vi "Main UI.vi"() -> ()   [LabVIEW 2017, in "Example UI.lvlib"]
uses:
  Example UI.lvlib
  CBTF Modules/Classes/Application/Class/typedefs/Test Info -- Cluster.ctl
  <vilib>/TSS/ACRObat Test Framework/Core Launcher/Core Manager Methods -- Enum.ctl
  <vilib>/TSS/ACRObat Test Framework/Utilities/User Manager/User Manager.Base/typedefs/User Groups -- Enum.ctl
  <vilib>/TSS/ACRObat Test Framework/Classes/Data/Data Viewer/Class/Data Viewer.lvclass
  C:/Program Files (x86)/National Instruments/LabVIEW 2017/vi.lib/TSS/ACRObat Test Framework/Classes/Base Objects/Base Class/Base Class/Base Class.lvclass
  CBTF Modules/Classes/Application/Class/typedefs/Op Mode -- Enum.ctl
  Application/Class/Example Application.lvclass
  C:/Test System Services/Acrobat Framework/CBTF Modules/Classes/Application/Class/Application.lvclass
  <vilib>/Utility/miscctls.llb/LVRowAndColumnTypeDef.ctl
  Application/Properties/DUT State -- Enum.ctl
  CBTF Modules/Classes/Test Recipe/Class/Test Recipe.lvclass
  CBTF Modules/Classes/Application/Class/Public API/Settings/Adjust Application Settings.vi
  <vilib>/TSS/ACRObat Test Framework/Utilities/User Manager/User Manager.FileDB/User Library.FileDB.lvclass
  <vilib>/TSS/ACRObat Test Framework/Classes/Data/Data Logger/Class/Data Logger.lvclass
  <vilib>/TSS/ACRObat Test Framework/Core Launcher/Core Launcher.lvlib
  <vilib>/TSS/ACRObat Test Framework/Classes/Base Objects/Base Class/Base Class/Base Class.lvclass
  CBTF Modules/Classes/Application/Class/Application.lvclass
  <vilib>/TSS/ACRObat Test Framework/Utilities/User Manager/User Manager.Base/User Library.Base.lvclass
  Application/Properties/Example App Properties.lvclass
  <vilib>/TSS/ACRObat Test Framework/Classes/Data/Data Repo/Class/Data Repo.lvclass
panel:
  out "Gold Board":bool
  in  "Iterations":u32=1
  in  "Serial 6":string caption="Serial ID 6"
  in  "Status 6":string
  in  "Serial 5":string caption="Serial ID 5"
  in  "Status 5":string
  in  "Serial 4":string caption="Serial ID 4"
  in  "Status 4":string
  in  "Settings":bool
  out "VER":bool
  out "ENG":bool
  in  "Serial 3":string caption="Serial ID 3"
  in  "Status 3":string
  in  "Serial 2":string caption="Serial ID 2"
  in  "Status 2":string
  in  "Serial 1":string caption="Serial ID 1"
  in  "Status 1":string
  in  "User Login":bool
  out "Results":i32(listbox)=-1
  in  "Test Information":T1
  in  "Run":bool
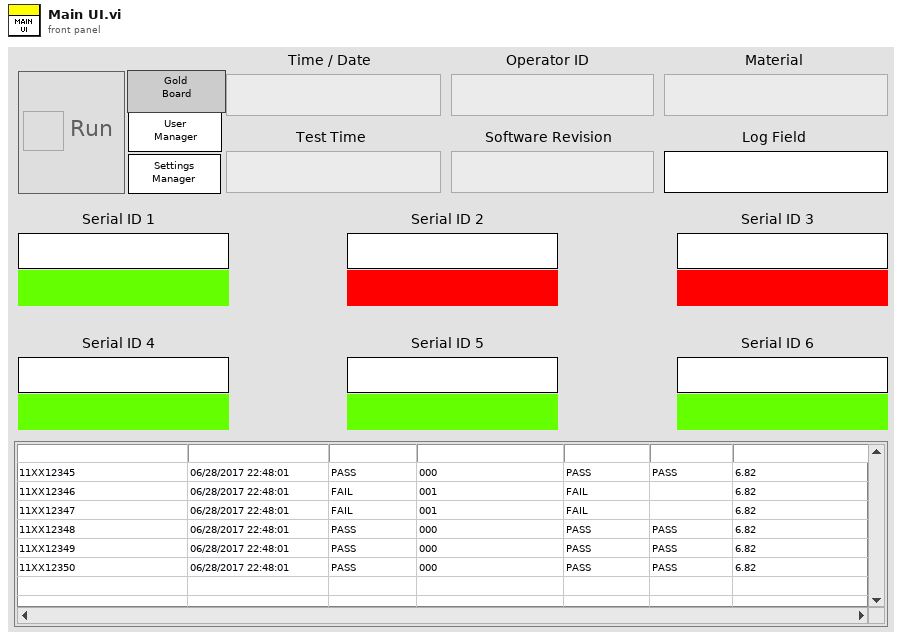
[diagram p1: front panel]
types:
  T1 = typedef "Application.lvlib/Application.lvclass/Test Info -- Cluster.ctl" = cluster{"Time / Date":string, "Operator ID":string, "Material":string, "Log Field":string, "Test Time":string, "Software Revision":string}
  T2 = typedef "Core Launcher.lvlib/Core Manager Methods -- Enum.ctl" = enum16{"Spawn Objects", "Get Objects", "Destroy Objects"}
  T3 = typedef "Utilities.lvlib/User Library.Base.lvclass/User Groups -- Enum.ctl" = enum16{"unknown", "Standard", "Engineering", "Super"}
  T4 = enum32{"invalid app kind", "Development System", "Run Time System", "Student Edition", "Embedded LabVIEW", "Evaluation", "Custom"}
  T5 = typedef "LVRowAndColumnTypeDef.ctl" = cluster{"Row":i32, "Column":i32}
  T6 = enum8{"Enabled", "Disabled", "Disabled and Grayed Out"}
  T7 = enum32{"Invalid", "Standard", "Closed", "Hidden", "Minimized", "Maximized"}
  T8 = enum16{"Idle", "Ready", "Running Test", "Paused"}
  T9 = typedef "Example Application.lvlib/Example App Properties.lvclass/DUT State -- Enum.ctl" = enum16{"Idle", "Ready", "Testing", "Passed", "Failed"}
  T10 = typedef "eventvkey.ctl" = enum16{"ASCII", "Enter", "Return", "Shift", "Ctrl", "Alt", "Cmd", "Opt", "Caps", "NumLock", "Clear", "Break", "Up", "Down", "Left", "Right", "Insert", "Delete", "Home", "End", "PageUp", "PageDown", "Escape", "Help", "Pause", "ScrollLock", "F1", "F2", "F3", "F4", "F5", "F6", "F7", "F8", "F9", "F10", "F11", "F12", "F13", "F14", "F15", "F16", "F17", "F18", "F19", "F20", "F21", "F22", "F23", "F24", "Play", "VolumeUp", "VolumeDown", "Mute", "Two Byte Char"}
  T11 = typedef "Application.lvlib/Application.lvclass/Op Mode -- Enum.ctl" = u16
  T12 = cluster{"Core":cluster{"Current VI Reference":refnum<vi>, "Close Panel on Exit?":bool}, "Application":refnum<class "Example Application.lvclass">, "Data Viewer":refnum<class "Data Viewer.lvclass">, "Op Mode":T11, "Current UUT":i16, "UI State":enum16{"Idle", "Ready", "Running Test", "Paused"}, "Tick Count":u64}
  T13 = cluster{"Current VI Reference":refnum<vi>, "Close Panel on Exit?":bool}
  T14 = typedef "Application.lvlib/App Properties.lvclass/Class Properties -- Cluster.ctl" = cluster{"UUT Info":T15[], "Test Information":refnum<vi>, "Gold Board":refnum<class "Golden Board.lvclass">, "Test Recipe":refnum<class "Test Recipe.lvclass">, "Instruments":refnum<class "Instrument.lvclass">[], "Mode":T11, "Test Results":T16[], "Station Config":refnum<class "Station Config.lvclass">, "Variable Engine":refnum<class "Variable Engine.lvclass">}
  T15 = typedef "Application.lvlib/App Properties.lvclass/UUT Reference -- Cluster.ctl" = cluster{"Serial Number Reference":refnum<vi>, "Status Message Reference":refnum<vi>}
  T16 = typedef "Application.lvlib/App Properties.lvclass/Test Result -- Cluster.ctl" = cluster{"Position":i32, "Pass":bool, "Fail Codes":string}
  T17 = typedef "Data Logger.lvlib/Data Logger Settings.lvclass/Class Settings -- Cluster.ctl" = cluster{"Mode":T18}
  T18 = typedef "Utilities.lvlib/DataLog Writer.lvclass/Data Mode -- Enum.ctl" = enum16{"Operator", "Engineering", "Verification"}
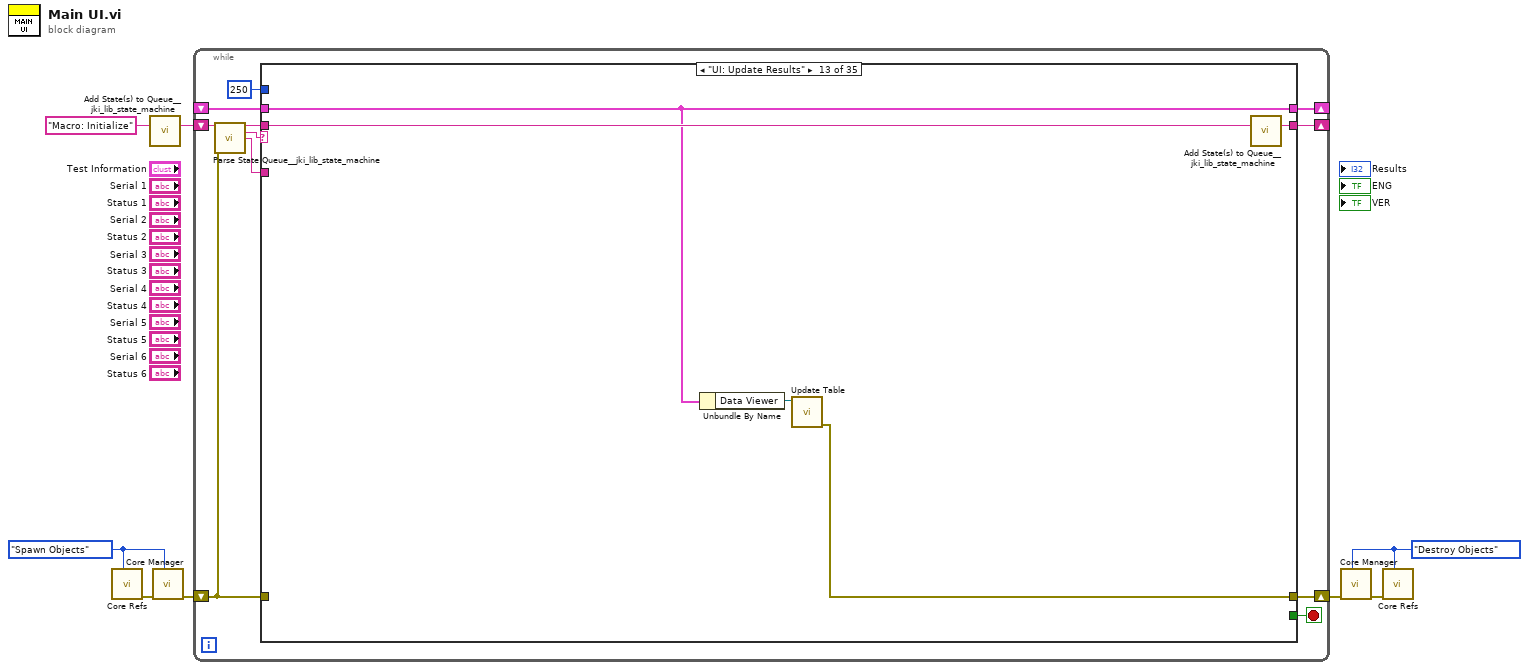
[diagram p0: block diagram]
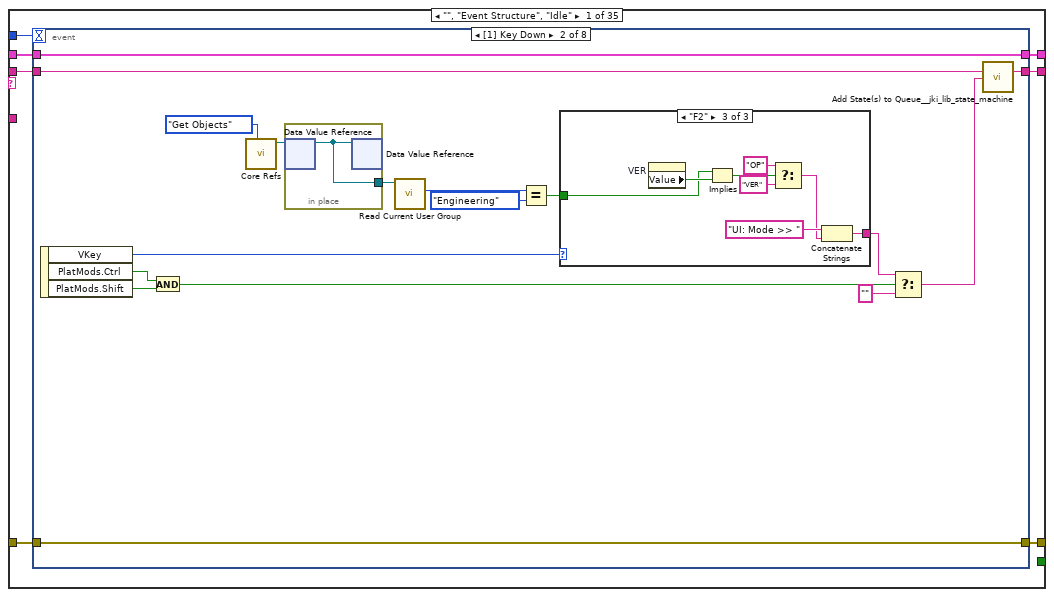
[diagram p2: hidden frame]
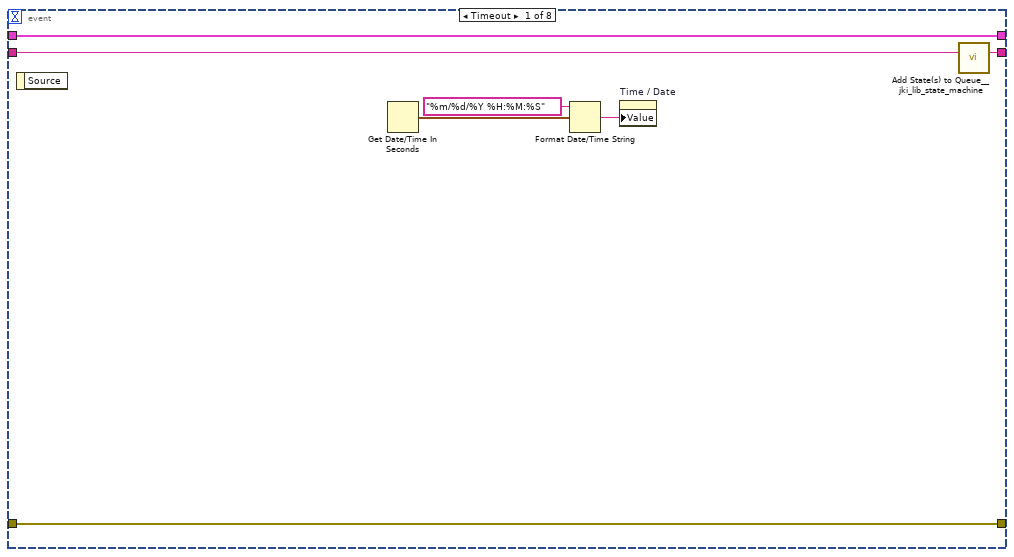
[diagram p3: hidden frame]
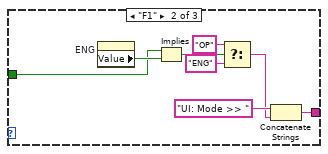
[diagram p5: hidden frame]
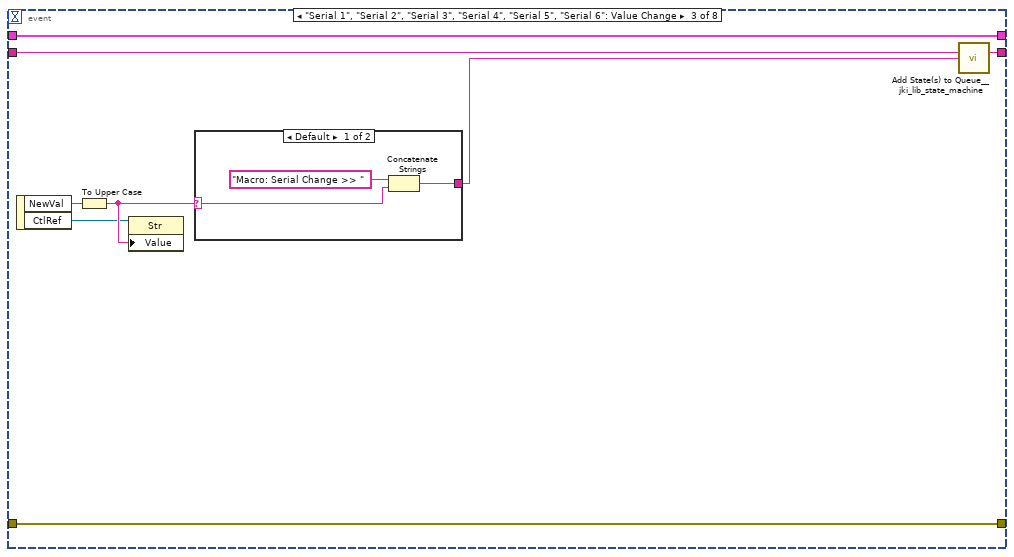
[diagram p6: hidden frame]
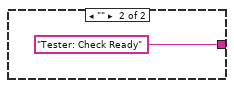
[diagram p7: hidden frame]
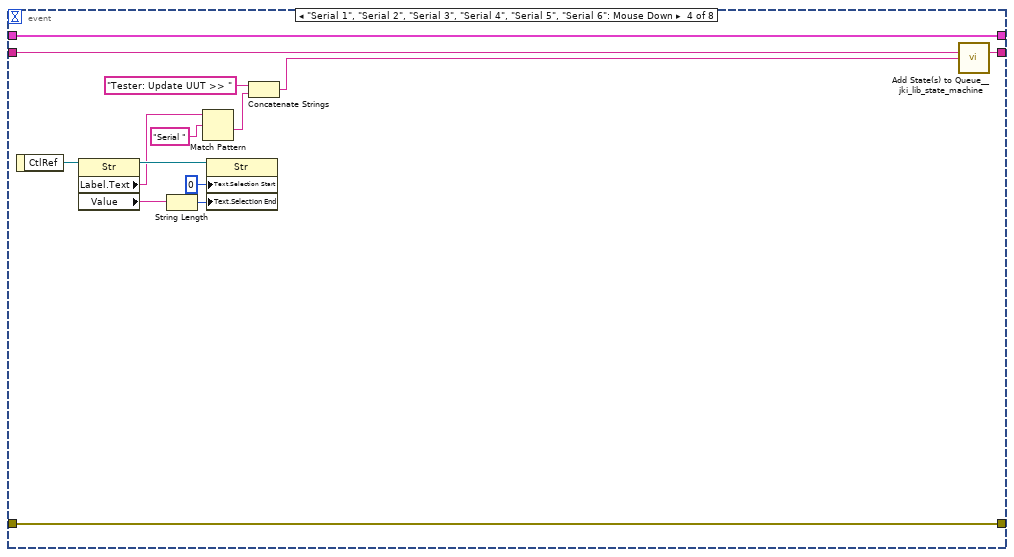
[diagram p8: hidden frame]
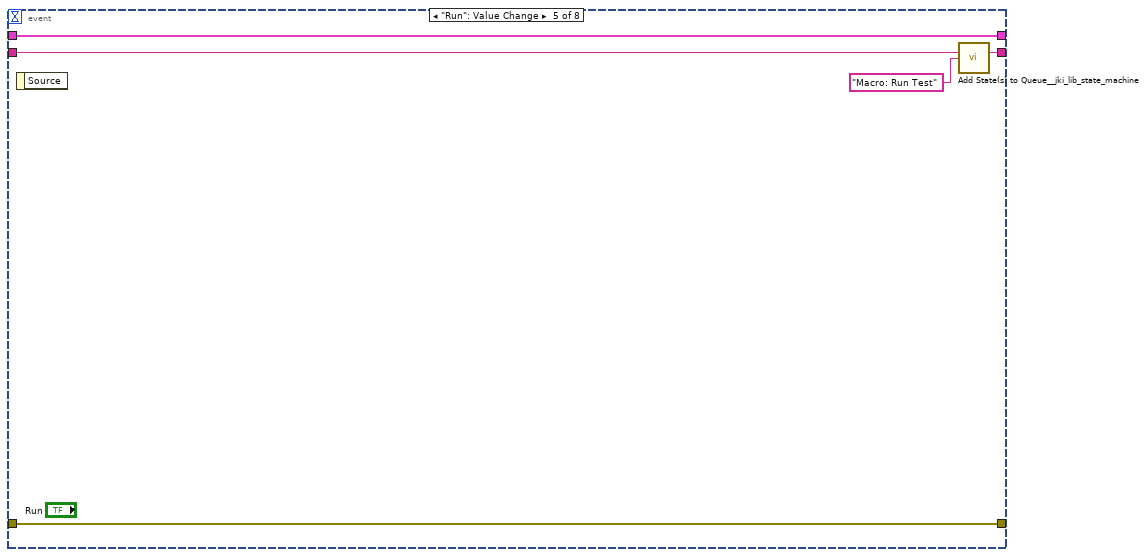
[diagram p9: hidden frame]
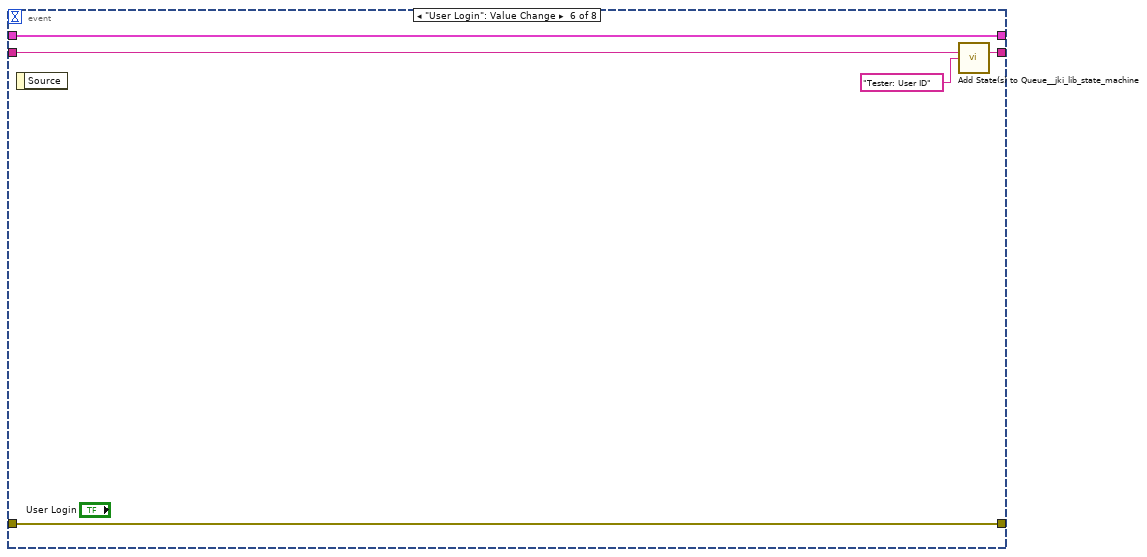
[diagram p10: hidden frame]
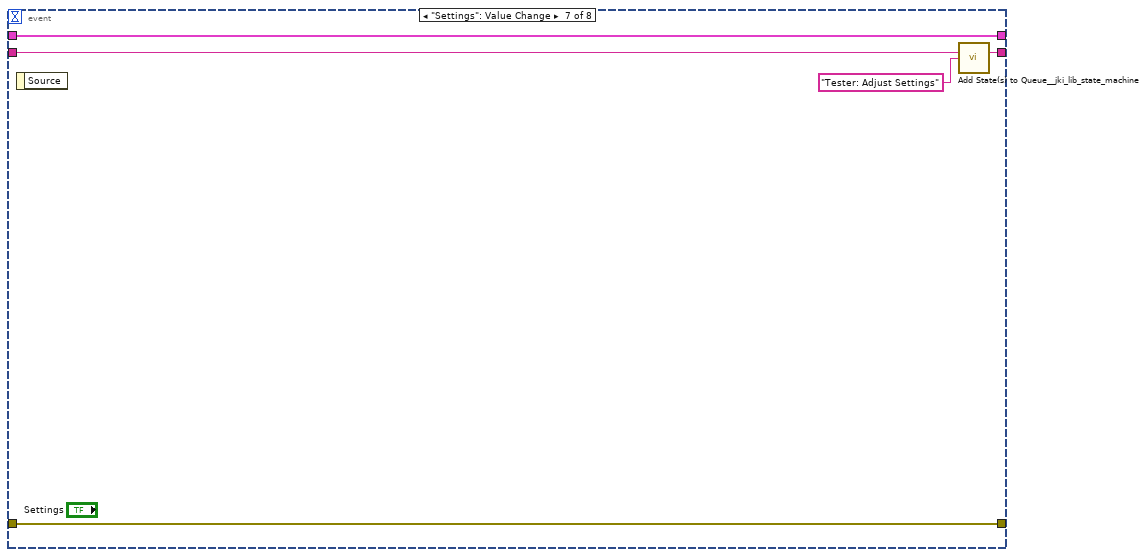
[diagram p11: hidden frame]
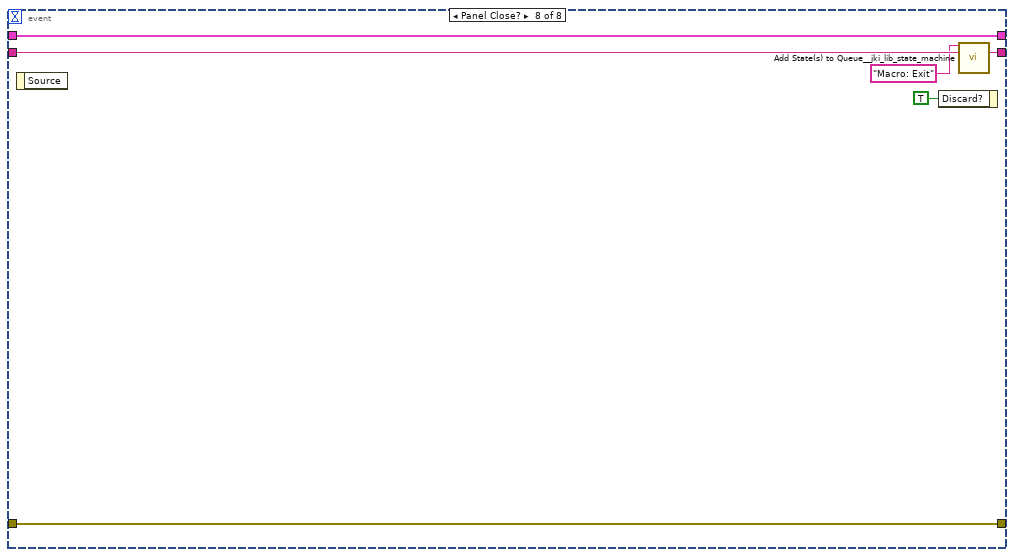
[diagram p12: hidden frame]
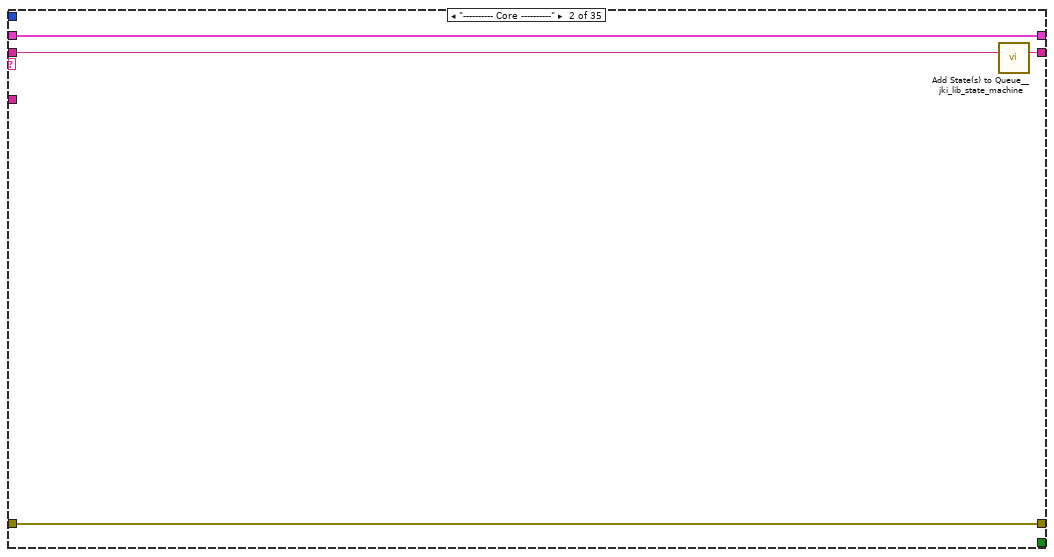
[diagram p13: hidden frame]
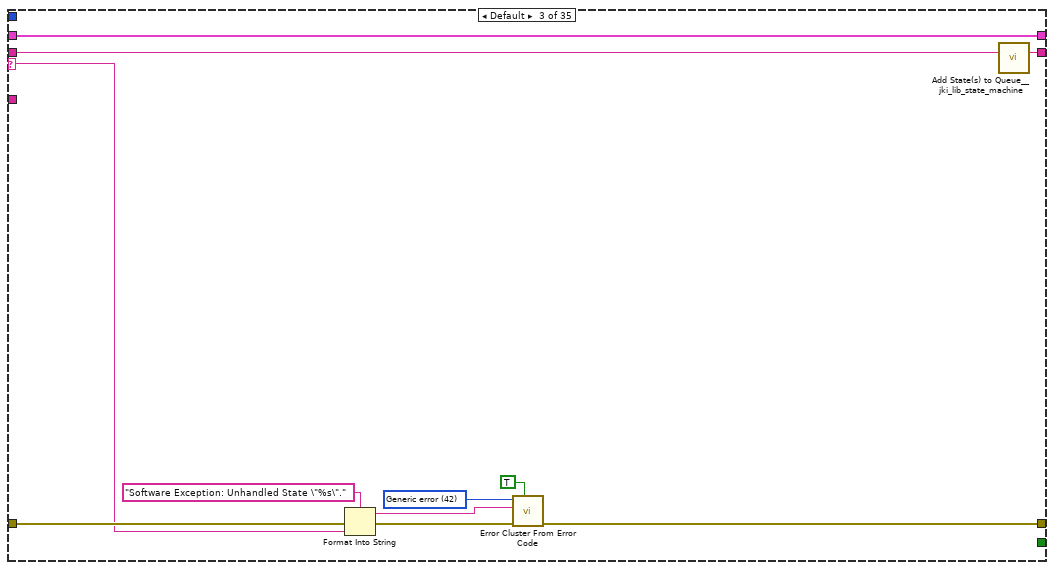
[diagram p14: hidden frame]
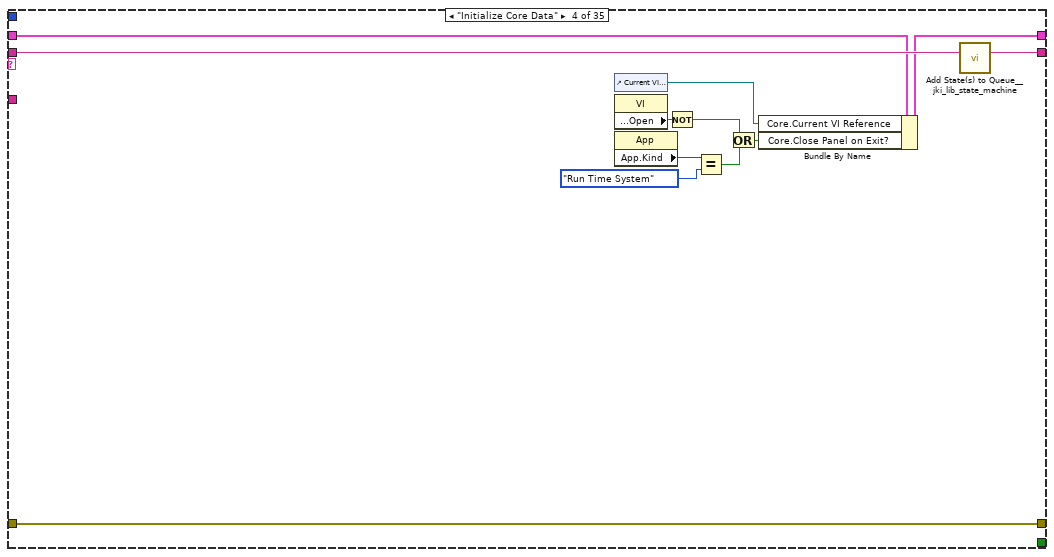
[diagram p15: hidden frame]
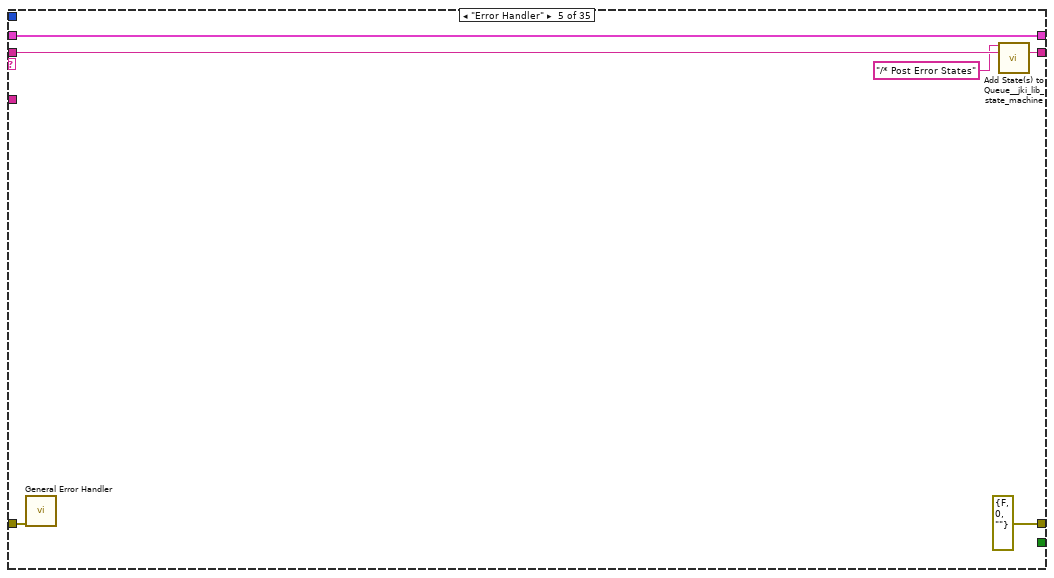
[diagram p16: hidden frame]
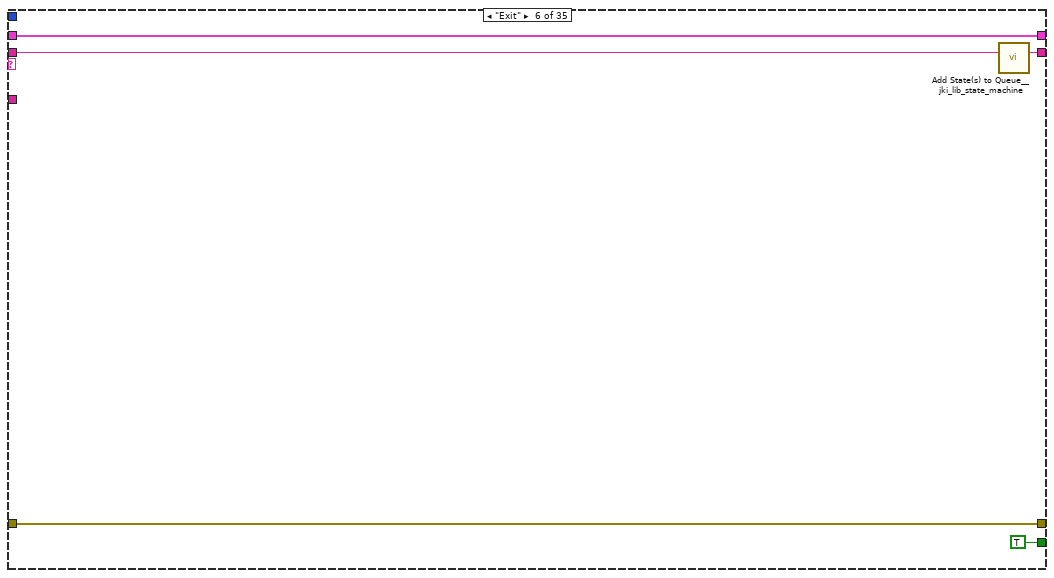
[diagram p17: hidden frame]
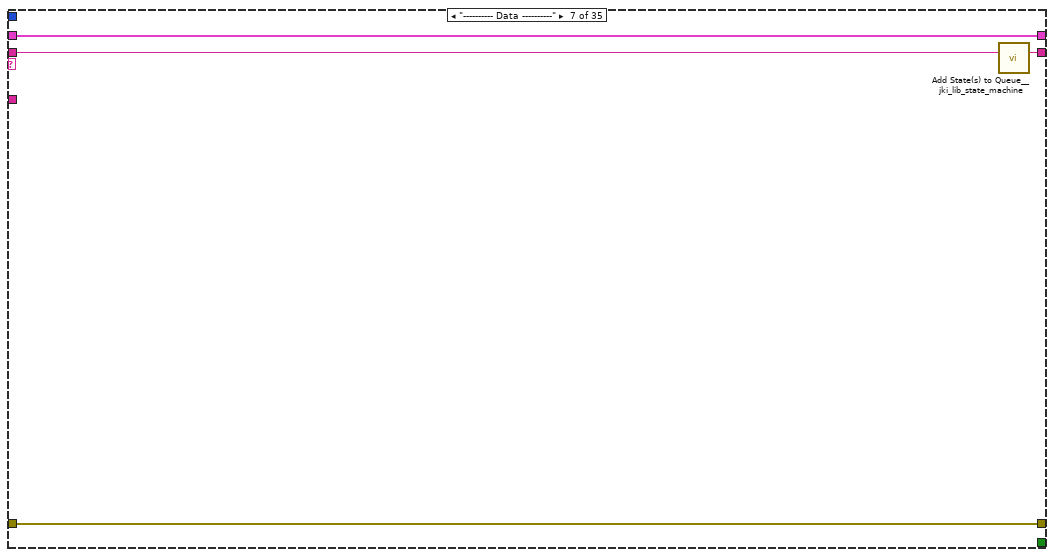
[diagram p18: hidden frame]
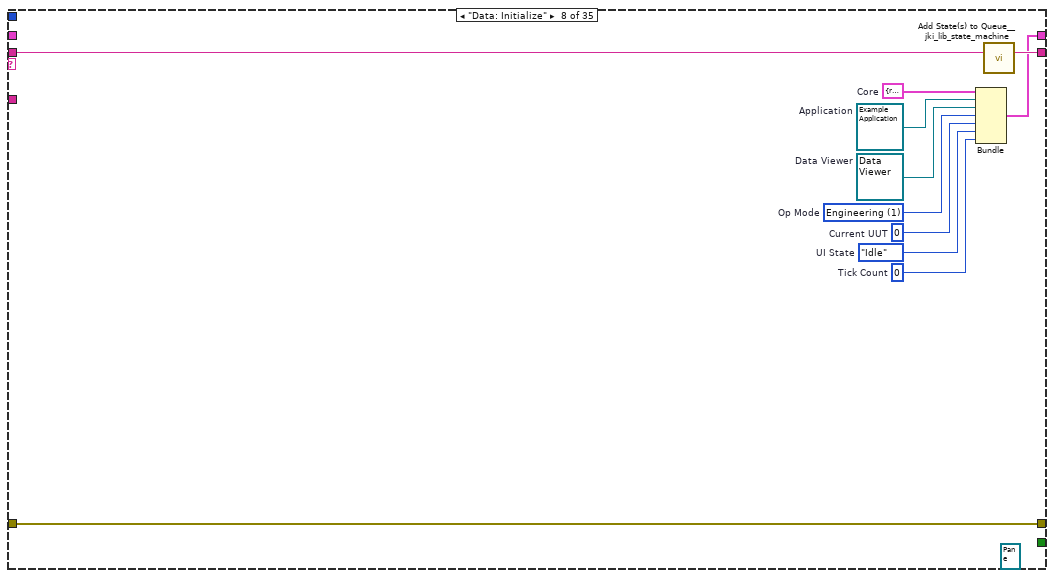
[diagram p19: hidden frame]
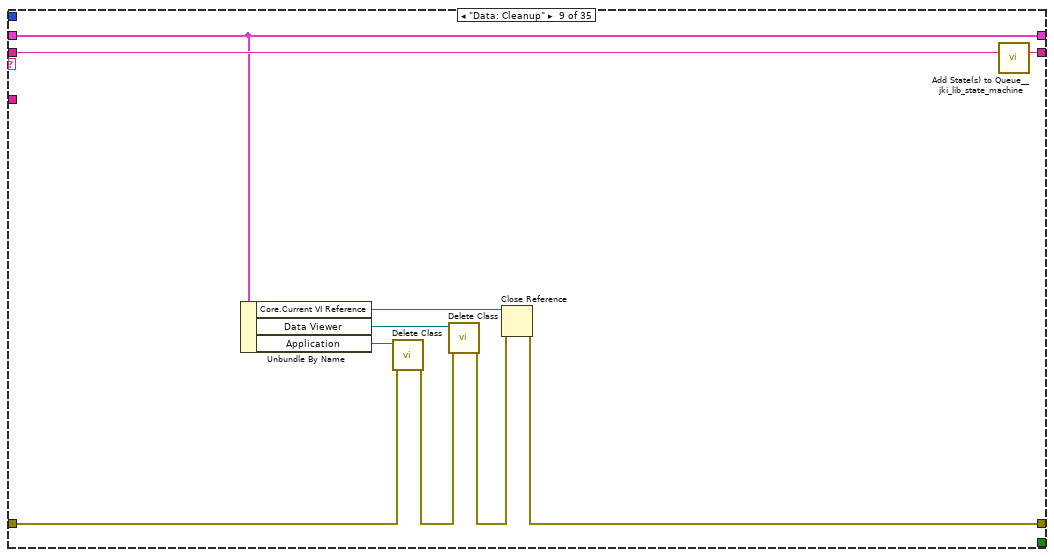
[diagram p20: hidden frame]
diagram:
  w7 = Core_Manager_Methods_--_Enum."Destroy Objects" ("Method")
  w5 = Core_Manager_Methods_--_Enum."Spawn Objects" ("Method")
  n1 = call <vilib>:"Core Refs.vi"("Method"=w5) -> ("error out"=w6:errorcluster)  [unwired: 8 in, 2 out]
  n2 = call <vilib>:"Add State(s) to Queue__jki_lib_state_machine.vi"("State(s) in (\"\")"="Macro: Initialize") -> ("States Out"=w4:string)  [unwired: 14 in]
  n3 = call <vilib>:"Core Manager.vi"("Method"=w5, "error in (no error)"=w6) -> ("error out"=w2:errorcluster)  [unwired: 5 in, 4 out]
  n4 = while {
    shift-right: [w13] -> _
    shift-left: _ -> [w12]
    shift-right: [w16] -> w1
    shift-left: w2 -> [w10]
    shift-right: [w15] -> _
    shift-left: w4 -> [w17]
    stop <- w14 stop-if-true
    n5 = call <vilib>:"Parse State Queue__jki_lib_state_machine.vi"("State Queue"=w17, "Error In (no error)"=w10) -> ("Remaining States"=w19:string, "Current State"=w9:string, "Arguments"=w18:string)  [unwired: 11 in]
    n6 = case shown="\"UI: Update Results\"" w9 {
      tunnel: w19 -> [w26 w118 w123 w141 w147 w152 w156 w167 w177 w181 w193 w205 w214 w236 w254 w273 w290 w311 w322 w348 w353 w360 w379 w387 w397 w401 w425 w433 w452 w459 w471 w487 w523 w547 w563]
      tunnel: w18 -> [_ _ _ _ _ _ _ _ _ _ _ _ _ w224 w248 w267 w285 w306 w316 _ _ _ _ w381 _ _ _ _ w443 w460 w466 _ _ _ _]
      tunnel: w12 -> [w24 w115 w121 w132 w144 w150 w153 _ w173 w178 w187 w196 w212 w227 w249 w268 w287 w309 w318 w345 w350 w357 w362 w384 w394 w398 w423 w431 w444 w457 w469 w473 w506 w526 w561]
      tunnel: [w23 w116 w125 w138 errorcluster {"status"=FALSE, "code"=0, "source"=""} ("error out") w149 w154 w164 w174 w179 w182 w195 w210 w225 w247 w266 w288 w307 w319 w346 w351 w358 w377 w385 w395 w399 w426 w427 w441 w453 w467 w485 w507 w527 w553] -> w16
      tunnel: w10 -> [w22 w116 w124 w138 w143 w149 w154 w164 w168 w179 _ _ _ _ _ _ w288 w308 w320 w346 w351 w358 w377 w385 w395 w399 _ _ _ w453 w467 w485 _ _ w553]
      tunnel: [w25 w117 w122 w140 w146 w151 w155 w166 w176 w180 w192 w204 w213 w235 w253 w272 w289 w310 w321 w347 w352 w359 w378 w386 w396 w400 w424 w432 w451 w458 w470 w486 w522 w546 w562] -> w15
      tunnel: [_ _ _ _ _ TRUE _ _ _ _ _ _ _ _ _ _ _ _ _ _ _ _ _ _ _ _ _ _ _ _ _ _ _ _ _] -> w14
      tunnel: [w21 w115 w121 w139 w144 w150 w153 w165 w173 w178 w187 w196 w212 w226 w249 w268 w287 w309 w318 w345 w350 w356 w361 w384 w394 w398 w416 w431 w444 w455 w468 w474 w520 w526 w561] -> w13
      tunnel: 250 ("Timeout") -> [w20 _ _ _ _ _ _ _ _ _ _ _ _ _ _ _ _ _ _ _ _ _ _ _ _ _ _ _ _ _ _ _ _ _ _]
      selector: w9 -> [_ _ w119 _ _ _ _ _ _ _ _ _ _ _ _ _ _ _ _ _ _ _ _ _ _ _ _ _ _ _ _ _ _ _ _]
      frame "", "Event Structure", "Idle" {
        n7 = event shown="[1] Key Down" {
          selector: _ -> [_ _ _ _ _ _ _ _]
          dyn-events: _ -> [_ _ _ _ _ _ _ _]
          timeout: w20 -> [_ _ _ _ _ _ _ _]
          tunnel: w26 -> [w33 w41 w75 w93 w98 w103 w108 w114]
          tunnel: [w32 w50 w74 w92 w97 w102 w107 w113] -> w25
          tunnel: w24 -> [w30 w40 w72 w90 w95 w100 w105 w111]
          tunnel: [w31 w49 w73 w91 w96 w101 w106 w112] -> w23
          tunnel: w22 -> [w31 w49 w73 w91 w96 w101 w106 w112]
          tunnel: [w30 w40 w72 w90 w95 w100 w105 w111] -> w21
          event Timeout {
            n8 = event-data() -> ()  [unwired: 1 in, 1 out]
            n9 = Get Date/Time In Seconds() -> (seconds since 1Jan1904=w29:timestamp)
            n10 = Format Date/Time String(time format string (%c)="%m/%d/%Y %H:%M:%S", seconds (now)=w29) -> (date/time string=w27:string)  [unwired: 1 in]
            n11 = property on="Time / Date" class="Str"("Value"=w27) -> ()  [unwired: 2 in, 2 out]
            n12 = call <vilib>:"Add State(s) to Queue__jki_lib_state_machine.vi"("State(s) in (\"\")"=w33) -> ("States Out"=w32:string)  [unwired: 14 in]
          }
          event Key Down {
            n13 = event-data() -> ("VKey"=w45:T10, "PlatMods.Ctrl"=w44:bool, "PlatMods.Shift"=w43:bool)  [unwired: 1 in]
            n14 = And(x=w44, y=w43) -> (x .and. y?=w46:bool)
            n15 = call <vilib>:"Core Refs.vi"("Method"=Core_Manager_Methods_--_Enum."Get Objects") -> ("User Manager Reference"=w38:refnum<data-value>)  [unwired: 8 in, 2 out]
            n16 = in-place {
              in-place-border: [w51] -> w37
              n17 = in-place-dvr #1(w38) -> (w51:refnum<class "User Library.FileDB.lvclass">)  [unwired: 1 out]
              n18 = in-place-dvr #1(w51) -> ()  [unwired: 2 out]
            }
            n19 = call-dynamic "Read Current User Group.vi"("User Manager in"=w37) -> ("Current User Group"=w36:T3)  [unwired: 8 in, 2 out]
            n20 = Equal?(x=w36, y=User_Groups_--_Enum."Engineering") -> (x = y?=w34:bool)
            n21 = case shown="\"F2\"" w45 {
              tunnel: [_ w56 w64] -> w48
              tunnel: w34 -> [_ w52 w60]
              frame Default {
              }
              frame "F1" {
                n22 = property on="ENG" class="Bool (strict)"() -> ("Value"=w53:bool)  [unwired: 2 in, 2 out]
                n23 = Implies(1:w53, 2:w52) -> (0:w54:bool)
                n24 = Select(t="OP", s=w54, f="ENG") -> (s? t:f=w55:string)
                n25 = Concatenate Strings("UI: Mode >> " ("State(s) at Back (\"\")"), w55) -> (w56:string)
              }
              frame "F2" {
                n26 = property on="VER" class="Bool (strict)"() -> ("Value"=w61:bool)  [unwired: 2 in, 2 out]
                n27 = Implies(1:w61, 2:w60) -> (0:w62:bool)
                n28 = Select(t="OP", s=w62, f="VER") -> (s? t:f=w63:string)
                n29 = Concatenate Strings("UI: Mode >> " ("State(s) at Back (\"\")"), w63) -> (w64:string)
              }
            }
            n30 = Select(t=w48, s=w46, f="" ("State(s) at Back (\"\")")) -> (s? t:f=w42:string)
            n31 = call <vilib>:"Add State(s) to Queue__jki_lib_state_machine.vi"("State(s) in (\"\")"=w41, "State(s) at Back (\"\")"=w42) -> ("States Out"=w50:string)  [unwired: 13 in]
          }
          event "Serial 1", "Serial 2", "Serial 3", "Serial 4", "Serial 5", "Serial 6": Value Change {
            n32 = event-data() -> ("NewVal"=w70:string, "CtlRef"=w69:refnum<vi>)  [unwired: 1 in]
            n33 = To Upper Case(1:w70) -> (0:w71:string)
            n34 = property class="Str"(reference=w69, "Value"=w71) -> ()  [unwired: 1 in, 2 out]
            n35 = case shown="Default" w71 {
              selector: w71 -> [w77 _]
              tunnel: [w76 "Tester: Check Ready"] -> w68
              frame Default {
                n36 = Concatenate Strings("Macro: Serial Change >> " ("State(s) at Back (\"\")"), w77) -> (w76:string)
              }
              frame "" {
              }
            }
            n37 = call <vilib>:"Add State(s) to Queue__jki_lib_state_machine.vi"("State(s) in (\"\")"=w75, "State(s) at Back (\"\")"=w68) -> ("States Out"=w74:string)  [unwired: 13 in]
          }
          event "Serial 1", "Serial 2", "Serial 3", "Serial 4", "Serial 5", "Serial 6": Mouse Down {
            n38 = event-data() -> ("CtlRef"=w85:refnum<vi>)  [unwired: 1 in]
            n39 = property class="Str"(reference=w85) -> (reference out=w86:refnum<vi>, "Label.Text"=w83:string, "Value"=w87:string)  [unwired: 1 in, 1 out]
            n40 = String Length(string=w87) -> (length=w89:i32)
            n41 = Match Pattern(string=w83, regular expression="Serial ") -> (after substring=w82:string)  [unwired: 1 in, 3 out]
            n42 = property class="Str"(reference=w86, "Text.Selection Start"=u32 0 ("Text.Selection:Start"), "Text.Selection End"=w89) -> ()  [unwired: 1 in, 2 out]
            n43 = Concatenate Strings("Tester: Update UUT >> ", w82) -> (w80:string)
            n44 = call <vilib>:"Add State(s) to Queue__jki_lib_state_machine.vi"("State(s) in (\"\")"=w93, "State(s) at Back (\"\")"=w80) -> ("States Out"=w92:string)  [unwired: 13 in]
          }
          event "Run": Value Change {
            n45 = event-data() -> ()  [unwired: 1 in, 1 out]
            n46 = call <vilib>:"Add State(s) to Queue__jki_lib_state_machine.vi"("State(s) in (\"\")"=w98, "State(s) at Back (\"\")"="Macro: Run Test" ("State(s) at Back (\"\")")) -> ("States Out"=w97:string)  [unwired: 13 in]
          }
          event "User Login": Value Change {
            n47 = event-data() -> ()  [unwired: 1 in, 1 out]
            n48 = call <vilib>:"Add State(s) to Queue__jki_lib_state_machine.vi"("State(s) in (\"\")"=w103, "State(s) at Back (\"\")"="Tester: User ID" ("State(s) at Back (\"\")")) -> ("States Out"=w102:string)  [unwired: 13 in]
          }
          event "Settings": Value Change {
            n49 = event-data() -> ()  [unwired: 1 in, 1 out]
            n50 = call <vilib>:"Add State(s) to Queue__jki_lib_state_machine.vi"("State(s) in (\"\")"=w108, "State(s) at Back (\"\")"="Tester: Adjust Settings" ("State(s) at Back (\"\")")) -> ("States Out"=w107:string)  [unwired: 13 in]
          }
          event Panel Close? {
            n51 = event-data() -> ()  [unwired: 1 in, 1 out]
            n52 = event-data("Discard?"=TRUE) -> ()  [unwired: 1 in, 1 out]
            n53 = call <vilib>:"Add State(s) to Queue__jki_lib_state_machine.vi"("State(s) in Front (\"\")"="Macro: Exit", "State(s) in (\"\")"=w114) -> ("States Out"=w113:string)  [unwired: 13 in]
          }
        }
      }
      frame "---------- Core ----------" {
        n54 = call <vilib>:"Add State(s) to Queue__jki_lib_state_machine.vi"("State(s) in (\"\")"=w118) -> ("States Out"=w117:string)  [unwired: 14 in]
      }
      frame Default {
        w128 = 42 items=["No error", "Argument error", "Memory is full", "Out of zone", "End of file", "File already open", "Generic file I/O error", "File not found", "File permission error", "Disk is full", "Duplicate path", "Too many files open", "System feature not enabled", "Resource file not found", "Cannot add resource", "Resource not found", "Image not found", "Image memory error", "Pen does not exist", "Config type invalid", "Config token not found", "Config parse error", "Config memory error", "Bad external code format", "Bad external code offset", "External code not present", "Null window", "Destroy window error", "Null menu", "Print aborted", "Bad print record", "Print driver error", "Windows error during printing", "Memory error during printing", "Print dialog error", "Generic print error", "Invalid device refnum", "Device not found", "Device parameter error", "Device unit error", "Cannot open device", "Device call aborted", "Generic error", "Cancelled by user", "Object ID too low", "Object ID too high", "Object not in heap", "Unknown heap", "Unknown object (invalid DefProc)", "Unknown object (DefProc not in table)", "Message out of range", "Invalid (null) method", "Unknown message", "Manager call not supported", "Bad address", "Network operation in progress", "Network operation timed out", "Connection is busy", "Network attribute not supported", "Network error", "Address in use", "System out of memory", "Connection aborted", "Connection refused", "Not connected", "Already connected", "Connection closed", "Initialization error (interapplication manager)", "Bad occurrence", "Wait on unbound occurrence handler", "Occurrence queue overflow", "Datalog type conflict", "Unused", "Unrecognized type (interapplication manager)", "Memory corrupt", "Failed to make temporary DLL", "Old CIN version", "Drag socket not found", "Failed to load drop-object", "Failed to register OLE object", "Failed to release OLE object", "Format specifier type mismatch", "Unknown format specifier", "Too few format specifiers", "Too many format specifiers", "Scan failed", "Newer CIN version", "Error converting to variant", "Runtime menu error", "Password tampered", "Variant attribute not found", "Incompatible variant data type", "Event data is not available", "Event Store is not present", "Occurrence is not found", "Event Queue is not created", "Event info is not available", "Refnum passed is NULL", "Error retrieving Class GUID", "Error retrieving CoClass GUID", "Error retrieving TypeLib GUID.", "Bad built application magic bytes.", "Specific driver is different from the specific driver associated with the Logical Name.", "There is no session opened to the class driver.", "Max Error", "MAX - Error with config objects", "MAX - Error loading configuration", "MAX - Group not supported"]
        n55 = Format Into String(format string="Software Exception: Unhandled State \"%s\"." ("message"), error in=w124, w119) -> (resulting string=w127:string, error out=w126:errorcluster)  [unwired: 1 in]
        n56 = call <vilib>:"Error Cluster From Error Code.vi"("show call chain? (False)"=TRUE, "error in (no error)"=w126, "error message (\"\")"=w127, "error code (0)"=w128) -> ("error out"=w125:errorcluster)  [unwired: 5 in]
        n57 = call <vilib>:"Add State(s) to Queue__jki_lib_state_machine.vi"("State(s) in (\"\")"=w123) -> ("States Out"=w122:string)  [unwired: 14 in]
      }
      frame "Initialize Core Data" {
        n58 = control-ref of="Current VI Reference"() -> (w130:refnum<vi>)
        n59 = property class="VI"() -> ("Front Panel.Open"=w137:bool)  [unwired: 2 in, 2 out]
        n60 = property class="App"() -> ("App.Kind"=w136:T4)  [unwired: 2 in, 2 out]
        n61 = Not(x=w137) -> (.not. x?=w134:bool)
        n62 = Equal?(x=w136, y=T4."Run Time System" ("Application:Kind")) -> (x = y?=w133:bool)
        n63 = Or(x=w134, y=w133) -> (x .or. y?=w131:bool)
        n64 = Bundle By Name(cluster=w132, "Core.Current VI Reference"=w130, "Core.Close Panel on Exit?"=w131) -> (w139:T12)
        n65 = call <vilib>:"Add State(s) to Queue__jki_lib_state_machine.vi"("State(s) in (\"\")"=w141) -> ("States Out"=w140:string)  [unwired: 14 in]
      }
      frame "Error Handler" {
        n66 = call <vilib>:"General Error Handler.vi"("error in (no error)"=w143) -> ()  [unwired: 10 in, 5 out]
        n67 = call <vilib>:"Add State(s) to Queue__jki_lib_state_machine.vi"("State(s) in Front (\"\")"="/* Post Error States", "State(s) in (\"\")"=w147) -> ("States Out"=w146:string)  [unwired: 13 in]
      }
      frame "Exit" {
        n68 = call <vilib>:"Add State(s) to Queue__jki_lib_state_machine.vi"("State(s) in (\"\")"=w152) -> ("States Out"=w151:string)  [unwired: 14 in]
      }
      frame "---------- Data ----------" {
        n69 = call <vilib>:"Add State(s) to Queue__jki_lib_state_machine.vi"("State(s) in (\"\")"=w156) -> ("States Out"=w155:string)  [unwired: 14 in]
      }
      frame "Data: Initialize" {
        w157 = u64 0  # Tick Count
        w158 = refnum<class "Example Application.lvclass"> refnum  # Application
        w159 = T11 1 items=["Operator", "Engineering", "Verification"]  # Op Mode
        w160 = T8."Idle"  # UI State
        w161 = refnum<class "Data Viewer.lvclass"> refnum  # Data Viewer
        (unwired) refnum<event-registration> refnum ("Event Registration Refnum")
        w162 = i16 0  # Current UUT
        w163 = T13 {"Current VI Reference"=refnum, "Close Panel on Exit?"=FALSE}  # Core
        n70 = Bundle("Core"=w163, "Application"=w158, "Data Viewer"=w161, "Op Mode"=w159, "Current UUT"=w162, "UI State"=w160, "Tick Count"=w157) -> (w165:T12)  [unwired: 1 in]
        n71 = call <vilib>:"Add State(s) to Queue__jki_lib_state_machine.vi"("State(s) in (\"\")"=w167) -> ("States Out"=w166:string)  [unwired: 14 in]
      }
      frame "Data: Cleanup" {
        n72 = Unbundle By Name(w173) -> ("Core.Current VI Reference"=w175:refnum<vi>, "Data Viewer"=w172:refnum<class "Data Viewer.lvclass">, "Application"=w170:refnum<class "Example Application.lvclass">)
        n73 = call <vilib>:"Delete Class.vi"("error in (no error)"=w168, "Base Class in"=w170) -> ("error out"=w169:errorcluster)  [unwired: 8 in, 1 out]
        n74 = call <vilib>:"Delete Class.vi"("error in (no error)"=w169, "Base Class in"=w172) -> ("error out"=w171:errorcluster)  [unwired: 8 in, 1 out]
        n75 = Close Reference(reference=w175, error in (no error)=w171) -> (error out=w174:errorcluster)
        n76 = call <vilib>:"Add State(s) to Queue__jki_lib_state_machine.vi"("State(s) in (\"\")"=w177) -> ("States Out"=w176:string)  [unwired: 14 in]
      }
      frame "---------- UI ----------" {
        n77 = call <vilib>:"Add State(s) to Queue__jki_lib_state_machine.vi"("State(s) in (\"\")"=w181) -> ("States Out"=w180:string)  [unwired: 14 in]
      }
      frame "UI: Initialize" {
        n78 = control-ref of="This VI"() -> (w191:refnum<vi>)
        n79 = invoke class="VI" method="Default Vals.Reinit All"(reference=w191) -> (error out=w194:errorcluster)  [unwired: 2 in, 2 out]
        n80 = call "Get App Version.vi"() -> ("error out"=w182:errorcluster, "Version"=w184:string)  [unwired: 10 in]
        n81 = property on="Results" class="MCListbox (strict)"(error in=w194, "ActiveCell"=T5 {"Row"=-2, "Column"=-2} ("Active Cell:Active Cell"), "CellBG"=u32 16777226, "ItemNames"=string[][] [] ("Item Names")) -> ()  [unwired: 1 in, 2 out]
        n82 = property on="Test Time" class="Str"(error in=w194, "Value"="0.000" ("Serial 1")) -> ()  [unwired: 1 in, 2 out]
        n83 = property on="ENG" class="Bool (strict)"(error in=w194, "Visible"=FALSE) -> ()  [unwired: 1 in, 2 out]
        n84 = property on="VER" class="Bool (strict)"(error in=w194, "Visible"=FALSE) -> ()  [unwired: 1 in, 2 out]
        n85 = property on="Software Revision" class="Str"(error in=w194, "Value"=w184) -> ()  [unwired: 1 in, 2 out]
        n86 = call <vilib>:"Add State(s) to Queue__jki_lib_state_machine.vi"("State(s) in (\"\")"=w193) -> ("States Out"=w192:string)  [unwired: 14 in]
      }
      frame "UI: Key Focus" {
        n87 = Unbundle By Name(w196) -> ("Application"=w202:refnum<class "Example Application.lvclass">, "Current UUT"=w198:i16)
        n88 = call "Get Properties.vi"("Acrobat Template in"=w202) -> ("Class Properties"=w201:T14)  [unwired: 8 in, 2 out]
        n89 = Unbundle By Name(w201) -> ("UUT Info"=w200:T15[])
        n90 = Array Size(array=w200) -> (size(s)=w199:i32)
        n91 = Less?(x=w198, y=w199) -> (x < y?=w197:bool)
        n92 = Index Array(array=w200, index=w198) -> (element=w203:T15)
        n93 = case shown="True" w197 {
          tunnel: w203 -> [_ w207]
          tunnel: [_ w208] -> w195
          frame False {
          }
          frame True {
            n94 = Unbundle By Name(w207) -> ("Serial Number Reference"=w206:refnum<vi>)
            n95 = property on="Property Node" class="Str"(reference=w206, "Key Focus"=TRUE) -> (error out=w208:errorcluster)  [unwired: 1 in, 1 out]
          }
        }
        n96 = call <vilib>:"Add State(s) to Queue__jki_lib_state_machine.vi"("State(s) in (\"\")"=w205) -> ("States Out"=w204:string)  [unwired: 14 in]
      }
      frame "UI: Update Results" {
        n97 = Unbundle By Name(w212) -> ("Data Viewer"=w211:refnum<class "Data Viewer.lvclass">)
        n98 = call <vilib>:"Update Table.vi"("Data Viewer in"=w211) -> ("error out"=w210:errorcluster)  [unwired: 9 in, 1 out]
        n99 = call <vilib>:"Add State(s) to Queue__jki_lib_state_machine.vi"("State(s) in (\"\")"=w214) -> ("States Out"=w213:string)  [unwired: 14 in]
      }
      frame "UI: Mode" {
        n100 = case shown="\"ver\"" w224 {
          tunnel: [w240 w243 w246] -> w222
          tunnel: [w240 w243 w246] -> w221
          tunnel: [w238 w242 w244] -> w220
          tunnel: [w238 w242 w244] -> w219
          tunnel: [w239 w241 w245] -> w218
          tunnel: [w239 w241 w245] -> w217
          tunnel: [FALSE w241 _] -> w215
          frame "op", Default {
            w238 = FALSE
            w239 = FALSE
            w240 = T11 0 items=["Operator", "Engineering", "Verification"] ("Mode")
          }
          frame "eng" {
            w242 = FALSE
            w241 = TRUE
            w243 = T11 1 items=["Operator", "Engineering", "Verification"] ("Mode")
          }
          frame "ver" {
            w244 = TRUE
            w245 = FALSE
            w246 = T11 2 items=["Operator", "Engineering", "Verification"] ("Mode")
          }
        }
        n101 = property on="VER" class="Bool (strict)"("Value"=w220, "Visible"=w219) -> ()  [unwired: 2 in, 2 out]
        n102 = property on="ENG" class="Bool (strict)"("Value"=w218, "Visible"=w217) -> ()  [unwired: 2 in, 2 out]
        n103 = Bundle By Name(cluster=w227, "Op Mode"=w221) -> (w226:T12)
        n104 = property on="Iterations" class="DigNum (strict)"("Visible"=w215, "Value"=u32 1 ("Iterations")) -> ()  [unwired: 2 in, 2 out]
        n105 = call <vilib>:"Core Manager.vi"("Method"=Core_Manager_Methods_--_Enum."Get Objects") -> ("DataLogger"=w232:refnum<class "Data Logger.lvclass">)  [unwired: 6 in, 4 out]
        n106 = call-dynamic "Get Data Log Settings.vi"("DataLogger in"=w232) -> ("error out"=w234:errorcluster, "Class Settings"=w223:T17, "DataLogger out"=w231:refnum<class "Data Logger.lvclass">)  [unwired: 8 in]
        n107 = Bundle By Name(cluster=w223, "Mode"=w222) -> (w230:T17)
        n108 = call-dynamic "Set Data Log Settings.vi"("error in (no error)"=w234, "Class Settings"=w230, "DataLogger in"=w231) -> ("error out"=w229:errorcluster, "DataLogger out"=w228:refnum<class "Data Logger.lvclass">)  [unwired: 7 in]
        n109 = call-dynamic "Initialize Data Log Writer.vi"("error in (no error)"=w229, "DataLogger in"=w228) -> ("error out"=w225:errorcluster)  [unwired: 8 in, 1 out]
        n110 = call <vilib>:"Add State(s) to Queue__jki_lib_state_machine.vi"("State(s) in (\"\")"=w236) -> ("States Out"=w235:string)  [unwired: 14 in]
      }
      frame "UI: Clear Serial" {
        n111 = Unbundle By Name(w249) -> ("Application"=w250:refnum<class "Example Application.lvclass">)
        n112 = call "Get Properties.vi"("Acrobat Template in"=w250) -> ("Class Properties"=w252:T14)  [unwired: 8 in, 2 out]
        n113 = Unbundle By Name(w252) -> ("UUT Info"=w251:T15[])
        n114 = for {
          tunnel: w251 -> [w257] mode=indexing
          tunnel: w248 -> [w265]
          shift-right: [w259] -> w247
          shift-left: _ -> [w258]
          n115 = Unbundle By Name(w257) -> ("Serial Number Reference"=w256:refnum<vi>)
          n116 = property class="Str"(reference=w256, error in=w258) -> (reference out=w261:refnum<vi>, error out=w255:errorcluster, "Value"=w263:string)
          n117 = Equal?(x=w265, y=w263) -> (x = y?=w264:bool)
          n118 = Select(t="", s=w264, f=w263) -> (s? t:f=w260:string)
          n119 = property class="Str"(reference=w261, error in=w255, "Value"=w260) -> (error out=w259:errorcluster)  [unwired: 1 out]
        }
        n120 = call <vilib>:"Add State(s) to Queue__jki_lib_state_machine.vi"("State(s) in (\"\")"=w254) -> ("States Out"=w253:string)  [unwired: 14 in]
      }
      frame "UI: Serial Controls" {
        n121 = Unbundle By Name(w268) -> ("Application"=w269:refnum<class "Example Application.lvclass">)
        n122 = call "Get Properties.vi"("Acrobat Template in"=w269) -> ("Class Properties"=w271:T14)  [unwired: 8 in, 2 out]
        n123 = Unbundle By Name(w271) -> ("UUT Info"=w270:T15[])
        n124 = for {
          tunnel: w270 -> [w284] mode=indexing
          tunnel: w267 -> [w283]
          shift-right: [w278] -> w266
          shift-left: _ -> [w277]
          n125 = To Lower Case(string=w283) -> (all lower case string=w282:string)
          n126 = Unbundle By Name(w284) -> ("Serial Number Reference"=w279:refnum<vi>)
          n127 = Equal?(x=w282, y="enable") -> (x = y?=w280:bool)
          n128 = Select(t=T6."Enabled" ("Disabled"), s=w280, f=T6."Disabled and Grayed Out" ("Disabled")) -> (s? t:f=w274:T6)
          n129 = property class="Str"(reference=w279, error in=w277, "DisabledEnum"=w274) -> (error out=w278:errorcluster)  [unwired: 1 out]
        }
        n130 = call <vilib>:"Add State(s) to Queue__jki_lib_state_machine.vi"("State(s) in (\"\")"=w273) -> ("States Out"=w272:string)  [unwired: 14 in]
      }
      frame "UI: Update" {
        n131 = Unbundle By Name(w287) -> ("Application"=w286:refnum<class "Example Application.lvclass">)
        n132 = case shown="\"Post-Test\"" w285 {
          tunnel: w286 -> [_ w295 _]
          frame Default {
          }
          frame "Post-Test" {
            n133 = control-ref of="Material"() -> (w293:refnum<vi>)
            n134 = call "Get Properties.vi"("Acrobat Template in"=w295) -> ("Class Properties"=w294:T14)  [unwired: 8 in, 2 out]
            n135 = Unbundle By Name(w294) -> ("UUT Info"=w298:T15[])
            n136 = property class="Str"(reference=w293, "Value"="") -> (error out=w297:errorcluster)  [unwired: 1 in, 1 out]
            n137 = for {
              tunnel: w297 -> [_]
              tunnel: w298 -> [w301] mode=indexing
              n138 = Unbundle By Name(w301) -> ("Serial Number Reference"=w300:refnum<vi>)
              n139 = property class="Str"(reference=w300, "Value"="") -> ()  [unwired: 1 in, 2 out]
            }
            n140 = property on="Run" class="Bool"("DisabledEnum"=T6."Disabled and Grayed Out" ("Disabled")) -> ()  [unwired: 2 in, 2 out]
            n141 = property on="User Login" class="Bool"("DisabledEnum"=T6."Enabled" ("Disabled")) -> ()  [unwired: 2 in, 2 out]
            n142 = property on="Settings" class="Bool"("DisabledEnum"=T6."Enabled" ("Disabled")) -> ()  [unwired: 2 in, 2 out]
          }
          frame "Running" {
            n143 = property on="Run" class="Bool"("DisabledEnum"=T6."Disabled and Grayed Out" ("Disabled")) -> ()  [unwired: 2 in, 2 out]
            n144 = property on="User Login" class="Bool"("DisabledEnum"=T6."Disabled and Grayed Out" ("Disabled")) -> ()  [unwired: 2 in, 2 out]
            n145 = property on="Settings" class="Bool"("DisabledEnum"=T6."Disabled and Grayed Out" ("Disabled")) -> ()  [unwired: 2 in, 2 out]
          }
        }
        n146 = call <vilib>:"Add State(s) to Queue__jki_lib_state_machine.vi"("State(s) in (\"\")"=w290) -> ("States Out"=w289:string)  [unwired: 14 in]
      }
      frame "UI: Cursor Set" {
        n147 = case shown="\"Idle\", Default" w306 {
          tunnel: w308 -> [w313 w315]
          tunnel: [w312 w314] -> w307
          frame "Idle", Default {
            n148 = call <vilib>:"Unset Busy.vi"("error in (no error)"=w313) -> ("error out"=w312:errorcluster)  [unwired: 10 in]
          }
          frame "Busy" {
            n149 = call <vilib>:"Set Busy.vi"("error in (no error)"=w315) -> ("error out"=w314:errorcluster)  [unwired: 9 in, 1 out]
          }
        }
        n150 = call <vilib>:"Add State(s) to Queue__jki_lib_state_machine.vi"("State(s) in (\"\")"=w311) -> ("States Out"=w310:string)  [unwired: 14 in]
      }
      frame "UI: Front Panel State" {
        n151 = Unbundle By Name(w318) -> ("Core.Current VI Reference"=w317:refnum<vi>)
        n152 = case shown="\"Open\", Default" w316 {
          tunnel: w320 -> [w326 w339]
          tunnel: [w328 w340] -> w319
          tunnel: w317 -> [w327 w337]
          frame "Open", Default {
            n153 = property class="VI"(reference=w327, error in=w326) -> (reference out=w324:refnum<vi>, error out=w325:errorcluster, "Front Panel.Open"=w323:bool)
            n154 = case shown="False" w323 {
              tunnel: [w331 w334] -> w328
              tunnel: w325 -> [w330 w334]
              tunnel: w324 -> [w329 _]
              frame False {
                n155 = invoke class="VI" method="FP.Open"(reference=w329, error in=w330, "Activate"=TRUE, "State"=T7."Standard") -> (error out=w331:errorcluster)  [unwired: 1 in, 4 out]
              }
              frame True {
              }
            }
          }
          frame "Close" {
            n156 = property class="VI"(reference=w337, error in=w339) -> (reference out=w336:refnum<vi>, error out=w338:errorcluster, "Front Panel.Open"=w335:bool)
            n157 = case shown="True" w335 {
              tunnel: [w341 w344] -> w340
              tunnel: w338 -> [w341 w343]
              tunnel: w336 -> [_ w342]
              frame False {
              }
              frame True {
                n158 = invoke class="VI" method="FP.Close"(reference=w342, error in=w343) -> (error out=w344:errorcluster)  [unwired: 1 in, 2 out]
              }
            }
          }
        }
        n159 = call <vilib>:"Add State(s) to Queue__jki_lib_state_machine.vi"("State(s) in (\"\")"=w322) -> ("States Out"=w321:string)  [unwired: 14 in]
      }
      frame "---------- Macro ----------" {
        n160 = call <vilib>:"Add State(s) to Queue__jki_lib_state_machine.vi"("State(s) in (\"\")"=w348) -> ("States Out"=w347:string)  [unwired: 14 in]
      }
      frame "Macro: Initialize" {
        w349 = "Data: Initialize\nInitialize Core Data\nUI: Cursor Set >> Busy\nTester: Start Application\nUI: Mode >> Standard\nUI: Initialize\nUI: Serial Controls >> Enable\nTester: Check Ready\nUI: Front Panel State >> Open\nUI: Cursor Set >> Idle\nTester: User ID\nUI: Key Focus"  # Data: Initialize Initialize Core Data UI: Cursor Set >> Busy Tester: Start Application UI: Mode >> Standard UI: Initialize UI: Serial Controls >> Enable Tester: Check Ready UI: Front Panel State >> Open UI: Cursor Set >> Idle Tester: User ID UI: Key Focus
        n161 = call <vilib>:"Add State(s) to Queue__jki_lib_state_machine.vi"("State(s) in Front (\"\")"=w349, "State(s) in (\"\")"=w353) -> ("States Out"=w352:string)  [unwired: 13 in]
      }
      frame "Macro: Run Test" {
        n162 = Bundle By Name(cluster=w357, "UI State"=T8."Running Test") -> (w356:T12)
        n163 = call <vilib>:"Add State(s) to Queue__jki_lib_state_machine.vi"("State(s) in Front (\"\")"="UI: Update >> Running\nUI: Serial Controls >> Disable\nTester: Run Test", "State(s) in (\"\")"=w360) -> ("States Out"=w359:string)  [unwired: 13 in]
      }
      frame "Macro: Test Done" {
        n164 = Decrement(x="Iterations") -> (x-1=w365:u32)
        n165 = Greater Than 0?(x=w365) -> (x > 0?=w367:bool)
        n166 = Select(t=T8."Running Test" ("UI State"), s=w367, f=T8."Idle" ("UI State")) -> (s? t:f=w369:T8)
        n167 = Select(t=w365, s=w367, f=u32 1 ("t")) -> (s? t:f=w366:u32)
        n168 = property on="Iterations" class="DigNum (strict)"("Value"=w366) -> ()  [unwired: 2 in, 2 out]
        n169 = Bundle By Name(cluster=w362, "Current UUT"=i16 0 ("Current DUT"), "UI State"=w369) -> (w361:T12)
        n170 = Select(t="Idle\nMacro: Run Test", s=w367, f="UI: Serial Controls >> Enable\nUI: Update >> Post-Test\nUI: Key Focus") -> (s? t:f=w373:string)
        n171 = Concatenate Strings("Tester: Post Test\nUI: Update Results\n", w373) -> (w363:string)
        n172 = call <vilib>:"Add State(s) to Queue__jki_lib_state_machine.vi"("State(s) in Front (\"\")"=w363, "State(s) in (\"\")"=w379) -> ("States Out"=w378:string)  [unwired: 13 in]
      }
      frame "Macro: Serial Change" {
        n173 = Concatenate Strings("UI: Update >> Scanned\nTester: Check Serial >> ", w381, "\nTester: Check Ready\nUI: Key Focus" ("string")) -> (w380:string)
        n174 = call <vilib>:"Add State(s) to Queue__jki_lib_state_machine.vi"("State(s) in (\"\")"=w387, "State(s) at Back (\"\")"=w380) -> ("States Out"=w386:string)  [unwired: 13 in]
      }
      frame "Macro: Exit" {
        n175 = Unbundle By Name(w394) -> ("Core.Close Panel on Exit?"=w393:bool)
        n176 = Select(t="UI: Front Panel State >> Close", s=w393, f="") -> (s? t:f=w390:string)
        n177 = call <vilib>:"Add State(s) to Queue__jki_lib_state_machine.vi"("State(s) in (\"\")"=w390, "State(s) at Back (\"\")"="Data: Cleanup\nExit") -> ("States Out"=w388:string)  [unwired: 13 in]
        n178 = call <vilib>:"Add State(s) to Queue__jki_lib_state_machine.vi"("State(s) in Front (\"\")"=w388, "State(s) in (\"\")"=w397) -> ("States Out"=w396:string)  [unwired: 13 in]
      }
      frame "---------- Tester ----------" {
        n179 = call <vilib>:"Add State(s) to Queue__jki_lib_state_machine.vi"("State(s) in (\"\")"=w401) -> ("States Out"=w400:string)  [unwired: 14 in]
      }
      frame "Tester: Start Application" {
        n180 = control-ref of="Results"() -> (w402:refnum<vi>)
        n181 = control-ref of="Serial 1"() -> (w422:refnum<vi>)
        n182 = control-ref of="Serial 2"() -> (w421:refnum<vi>)
        n183 = control-ref of="Serial 3"() -> (w420:refnum<vi>)
        n184 = control-ref of="Serial 4"() -> (w415:refnum<vi>)
        n185 = control-ref of="Serial 5"() -> (w414:refnum<vi>)
        n186 = control-ref of="Serial 6"() -> (w413:refnum<vi>)
        n187 = control-ref of="Status 1"() -> (w419:refnum<vi>)
        n188 = control-ref of="Status 2"() -> (w418:refnum<vi>)
        n189 = control-ref of="Status 3"() -> (w417:refnum<vi>)
        n190 = control-ref of="Status 4"() -> (w412:refnum<vi>)
        n191 = control-ref of="Status 5"() -> (w411:refnum<vi>)
        n192 = control-ref of="Status 6"() -> (w410:refnum<vi>)
        n193 = control-ref of="Test Information"() -> (w407:refnum<vi>)
        n194 = Build Array(w422, w421, w420, w415, w414, w413) -> (w406:refnum<vi>[])
        n195 = Build Array(w419, w418, w417, w412, w411, w410) -> (w405:refnum<vi>[])
        n196 = call "Start User Interface for Application.vi"("Status References"=w405, "Serial References"=w406, "Test Information"=w407, "Name"="ExampleApplication", "Application in"=refnum<class "Example Application.lvclass"> refnum ("Example Application.lvlib:Example Application.lvclass")) -> ("error out"=w426:errorcluster, "Application out"=w404:refnum<class "Example Application.lvclass">)  [unwired: 5 in]
        n197 = call "Start Data Viewer.vi"("Results"=w402, "Application in"=w404) -> ("Data Viewer out"=w403:refnum<class "Data Viewer.lvclass">)  [unwired: 8 in, 1 out]
        n198 = Bundle By Name(cluster=w423, "Application"=w404, "Data Viewer"=w403) -> (w416:T12)
        n199 = call <vilib>:"Add State(s) to Queue__jki_lib_state_machine.vi"("State(s) in (\"\")"=w425) -> ("States Out"=w424:string)  [unwired: 14 in]
      }
      frame "Tester: User ID" {
        n200 = call <vilib>:"Core Refs.vi"("Method"=Core_Manager_Methods_--_Enum."Get Objects") -> ("User Manager Reference"=w429:refnum<data-value>)  [unwired: 8 in, 2 out]
        n201 = in-place {
          in-place-border: [w435] -> w428
          in-place-border: [w434] -> w427
          n202 = in-place-dvr #2(w429) -> (w437:refnum<class "User Library.FileDB.lvclass">)  [unwired: 1 out]
          n203 = call-dynamic "Login.vi"("User Manager in"=w437) -> ("error out"=w439:errorcluster, "User Manager out"=w438:refnum<class "User Library.FileDB.lvclass">)  [unwired: 9 in]
          n204 = call-dynamic "Read Current User.vi"("error in (no error)"=w439, "User Manager in"=w438) -> ("error out"=w434:errorcluster, "Current User"=w435:string, "User Manager out"=w436:refnum<class "User Library.FileDB.lvclass">)  [unwired: 7 in]
          n205 = in-place-dvr #2(w436) -> ()  [unwired: 2 out]
        }
        n206 = property on="Operator ID" class="Str"("Value"=w428) -> ()  [unwired: 2 in, 2 out]
        n207 = call <vilib>:"Add State(s) to Queue__jki_lib_state_machine.vi"("State(s) in (\"\")"=w433) -> ("States Out"=w432:string)  [unwired: 14 in]
      }
      frame "Tester: Check Serial" {
        n208 = control-ref of="Material"() -> (w442:refnum<vi>)
        n209 = Unbundle By Name(w444) -> ("Application"=w446:refnum<class "Example Application.lvclass">)
        n210 = property class="Str"(reference=w442) -> (reference out=w449:refnum<vi>, "Value"=w448:string)  [unwired: 1 in, 1 out]
        n211 = property on="ENG" class="Bool (strict)"() -> ("Value"=w447:bool)  [unwired: 2 in, 2 out]
        n212 = call "Get Material Name from Serial Number.vi"("Engineering Mode"=w447, "Material Type Reference"=w448, "Serial Number"=w443, "Application in"=w446) -> ("error out"=w441:errorcluster, "Material Type out"=w450:string, "Gold Board"=→"Gold Board":bool, "Next State"=w445:string)  [unwired: 4 in]
        n213 = property class="Str"(reference=w449, "Value"=w450) -> ()  [unwired: 1 in, 2 out]
        n214 = call <vilib>:"Add State(s) to Queue__jki_lib_state_machine.vi"("State(s) in Front (\"\")"=w445, "State(s) in (\"\")"=w452) -> ("States Out"=w451:string)  [unwired: 13 in]
      }
      frame "Tester: Increment UUT" {
        n215 = Unbundle By Name(w457) -> ("Current UUT"=w456:i16)
        n216 = case shown="Default" w460 {
          tunnel: w456 -> [w462 _]
          tunnel: [w461 _] -> w454
          frame Default {
            n217 = Increment(x=w462) -> (x+1=w461:i16)
          }
          frame "Reset" {
          }
        }
        n218 = Bundle By Name(cluster=w457, "Current UUT"=w454) -> (w455:T12)
        n219 = call <vilib>:"Add State(s) to Queue__jki_lib_state_machine.vi"("State(s) in (\"\")"=w459) -> ("States Out"=w458:string)  [unwired: 14 in]
      }
      frame "Tester: Update UUT" {
        n220 = Scan From String(input string=w466, default 1=i16 0 ("Current UUT")) -> (output 1=w464:i16)  [unwired: 3 in, 3 out]
        n221 = Decrement(x=w464) -> (x-1=w463:i16)
        n222 = Bundle By Name(cluster=w469, "Current UUT"=w463) -> (w468:T12)
        n223 = call <vilib>:"Add State(s) to Queue__jki_lib_state_machine.vi"("State(s) in (\"\")"=w471) -> ("States Out"=w470:string)  [unwired: 14 in]
      }
      frame "Tester: Check Ready" {
        n224 = Unbundle By Name(w473) -> ("Application"=w472:refnum<class "Example Application.lvclass">)
        n225 = call "Get Properties.vi"("Acrobat Template in"=w472) -> ("Class Properties"=w475:T14)  [unwired: 8 in, 2 out]
        n226 = Unbundle By Name(w475) -> ("UUT Info"=w484:T15[])
        n227 = for {
          tunnel: [w500] -> w479 mode=indexing
          tunnel: w484 -> [w497] mode=indexing
          tunnel: w472 -> [w494]
          i -> [w493]
          n228 = Unbundle By Name(w497) -> ("Status Message Reference"=w496:refnum<vi>, "Serial Number Reference"=w495:refnum<vi>)
          n229 = property class="Str"(reference=w495) -> ("Value"=w505:string)  [unwired: 1 in, 2 out]
          n230 = Empty String/Path?(string/path=w505) -> (empty?=w491:bool)
          n231 = Select(t="Scan Serial ID" ("Status"), s=w491, f="Ready" ("Status")) -> (s? t:f=w499:string)
          n232 = Select(t=u32 16777226, s=w491, f=u32 1245180) -> (s? t:f=w498:u32)
          n233 = Select(t=DUT_State_--_Enum."Idle" ("Enum"), s=w491, f=DUT_State_--_Enum."Ready" ("Enum")) -> (s? t:f=w488:T9)
          n234 = Not(x=w491) -> (.not. x?=w500:bool)
          n235 = property class="Str"(reference=w496, "Value"=w499, "Text.BGColor"=w498) -> ()  [unwired: 1 in, 2 out]
          n236 = Increment(x=w493) -> (x+1=w492:i32)
          n237 = call-dynamic "Set State by Position.vi"("State"=w488, "Position"=w492, "Example Application in"=w494) -> ()  [unwired: 7 in, 2 out]
        }
        n238 = Or Array Elements(Boolean array=w479) -> (logical OR=w483:bool)
        n239 = Select(t=T8."Ready" ("UI State"), s=w483, f=T8."Idle") -> (s? t:f=w476:T8)
        n240 = Select(t=T6."Enabled" ("Disabled"), s=w483, f=T6."Disabled and Grayed Out" ("Disabled")) -> (s? t:f=w480:T6)
        n241 = Bundle By Name(cluster=w473, "UI State"=w476) -> (w474:T12)
        n242 = property on="Run" class="Bool"("DisabledEnum"=w480) -> ()  [unwired: 2 in, 2 out]
        n243 = call <vilib>:"Add State(s) to Queue__jki_lib_state_machine.vi"("State(s) in (\"\")"=w487) -> ("States Out"=w486:string)  [unwired: 14 in]
      }
      frame "Tester: Run Test" {
        n244 = Unbundle By Name(w506) -> ("Application"=w510:refnum<class "Example Application.lvclass">)
        n245 = property on="Material" class="Str"() -> ("Value"=w509:string)  [unwired: 2 in, 2 out]
        n246 = call "Read Test Recipe.vi"("Test Recipe in"=refnum<class "Test Recipe.lvclass"> refnum ("Golden Board in"), "Material Type"=w509) -> ("Test Recipe out"=w511:refnum<class "Test Recipe.lvclass">)  [unwired: 8 in, 1 out]
        n247 = call "Set Recipe.vi"("Golden Board in"=w511, "Acrobat Template in"=w510) -> ("Acrobat Template out"=w512:refnum<class "Example Application.lvclass">)  [unwired: 8 in, 1 out]
        n248 = call "Set All Active UUTs to Testing.vi"("Application in"=w512) -> ("Number of Active DUTs"=w516:i32, "Application out"=w513:refnum<class "Example Application.lvclass">)  [unwired: 8 in, 1 out]
        n249 = call <vilib>:"Core Manager.vi"("Method"=Core_Manager_Methods_--_Enum."Get Objects") -> ("Data Repo"=w514:refnum<class "Data Repo.lvclass">)  [unwired: 6 in, 4 out]
        n250 = call "Display All Idle.vi"("Application in"=w513) -> ("Application out"=w517:refnum<class "Example Application.lvclass">)  [unwired: 9 in, 1 out]
        n251 = call <vilib>:"Initialize Data Repository.vi"("Number of DUTs"=w516, "Acrobat Template in"=w514) -> ("error out"=w518:errorcluster)  [unwired: 8 in, 1 out]
        n252 = call-dynamic "Run Test Application.vi"("error in (no error)"=w518, "Application Template in"=w517) -> ("error out"=w507:errorcluster)  [unwired: 8 in, 1 out]
        n253 = Tick Count (ms)() -> (millisecond timer value=w521:u32)
        n254 = Bundle By Name(cluster=w506, "Tick Count"=w521) -> (w520:T12)
        n255 = call <vilib>:"Add State(s) to Queue__jki_lib_state_machine.vi"("State(s) in (\"\")"=w523, "State(s) at Back (\"\")"="Macro: Test Done" ("State(s) at Back (\"\")")) -> ("States Out"=w522:string)  [unwired: 13 in]
      }
      frame "Tester: Post Test" {
        n256 = Unbundle By Name(w526) -> ("Tick Count"=w542:u64, "Application"=w524:refnum<class "Example Application.lvclass">)
        n257 = Tick Count (ms)() -> (millisecond timer value=w543:u32)
        n258 = Subtract(x=w543, y=w542) -> (x-y=w541:u64)
        n259 = call-dynamic "Post Test.vi"("Application in"=w524) -> ("error out"=w525:errorcluster)  [unwired: 9 in, 1 out]
        n260 = To Double Precision Float(number=w541) -> (double precision float=w539:dbl)
        n261 = call <vilib>:"Core Manager.vi"("Method"=Core_Manager_Methods_--_Enum."Get Objects") -> ("Data Repo"=w538:refnum<class "Data Repo.lvclass">)  [unwired: 6 in, 4 out]
        n262 = Divide(x=w539, y=1000.0) -> (x/y=w529:dbl)
        n263 = call <vilib>:"Get All Data.vi"("Acrobat Template in"=w538) -> ("Data"=w536:refnum<class "Dictionary.lvclass">[], "Acrobat Template out"=w537:refnum<class "Data Repo.lvclass">)  [unwired: 8 in, 1 out]
        n264 = Format Into String(format string="%.2f", w529) -> (resulting string=w528:string)  [unwired: 2 in, 1 out]
        n265 = Array Size(array=w536) -> (size(s)=w535:i32)
        n266 = for {
          N: w535 -> [_]
          tunnel: w537 -> [w552]
          tunnel: [w549] -> w534 mode=indexing
          tunnel: w528 -> [w548]
          i -> [w551]
          n267 = call <vilib>:"Set Data by Row.vi"("Row"=w551, "Value"=w548, "Header"="TestTime", "Acrobat Template in"=w552) -> ("error out"=w549:errorcluster)  [unwired: 6 in, 1 out]
        }
        n268 = property on="Test Time" class="Str"("Value"=w528) -> ()  [unwired: 2 in, 2 out]
        n269 = Merge Errors(w534) -> (w533:errorcluster)
        n270 = call <vilib>:"Core Manager.vi"("Method"=Core_Manager_Methods_--_Enum."Get Objects") -> ("DataLogger"=w531:refnum<class "Data Logger.lvclass">)  [unwired: 6 in, 4 out]
        n271 = call-dynamic "Write Results to File.vi"("error in (no error)"=w533, "DataLogger in"=w531) -> ("error out"=w544:errorcluster)  [unwired: 8 in, 1 out]
        n272 = Merge Errors(w544, w525) -> (w527:errorcluster)
        n273 = call <vilib>:"Add State(s) to Queue__jki_lib_state_machine.vi"("State(s) in (\"\")"=w547) -> ("States Out"=w546:string)  [unwired: 14 in]
      }
      frame "Tester: Adjust Settings" {
        n274 = call <vilib>:"Core Refs.vi"("Method"=Core_Manager_Methods_--_Enum."Get Objects") -> ("User Manager Reference"=w559:refnum<data-value>)  [unwired: 8 in, 2 out]
        n275 = in-place {
          in-place-border: [w569] -> w558
          n276 = in-place-dvr #3(w559) -> (w569:refnum<class "User Library.FileDB.lvclass">)  [unwired: 1 out]
          n277 = in-place-dvr #3(w569) -> ()  [unwired: 2 out]
        }
        n278 = Unbundle By Name(w561) -> ("Application"=w554:refnum<class "Example Application.lvclass">)
        n279 = call-dynamic "Read Current User Group.vi"("User Manager in"=w558) -> ("Current User Group"=w557:T3)  [unwired: 8 in, 2 out]
        n280 = Equal?(x=w557, y=User_Groups_--_Enum."Engineering") -> (x = y?=w555:bool)
        n281 = case shown="True" w555 {
          tunnel: w554 -> [_ w564]
          frame False {
          }
          frame True {
            n282 = vi-ref "Application.lvlib:Application.lvclass:Adjust Application Settings.vi"() -> (w567:refnum<vi>)
            n283 = property class="VI Interface Type 6"(reference=w567) -> ("Name"=w566:string)  [unwired: 1 in, 2 out]
            n284 = Open VI Reference(type specifier VI Refnum (for type only)=w567, vi path=w566, options=128) -> (vi reference=w565:refnum<vi>)  [unwired: 3 in, 1 out]
            n285 = call-by-ref "Start Asynchronous Call"(reference=w565, "Application in"=w564) -> ()  [unwired: 10 in, 4 out]
          }
        }
        n286 = call <vilib>:"Add State(s) to Queue__jki_lib_state_machine.vi"("State(s) in (\"\")"=w563) -> ("States Out"=w562:string)  [unwired: 14 in]
      }
    }
  }
  n287 = call <vilib>:"Core Manager.vi"("Method"=w7, "error in (no error)"=w1) -> ("error out"=w8:errorcluster)  [unwired: 5 in, 4 out]
  n288 = call <vilib>:"Core Refs.vi"("Method"=w7, "error in (no error)"=w8) -> ()  [unwired: 7 in, 3 out]
